vi "Discrete Integrator (DBL Array).vi"(2 "initialize":bool, 3 "initial conditions":dbl[](array[numeric]) format="%.2f", 5 "input points":dbl[](array[numeric]) format="%.2f") -> (1 "output points":dbl[](array[numeric]) format="%.2f")   [LabVIEW 2017, in "NI_AdvCtrl_discrete linear.lvlib"]
doc: "LabVIEW no longer supports this VI. You can obtain similar functionality by installing the LabVIEW Simulation Module.\n\nIntegrates a discrete input signal. The integration process is based on Euler method."
uses:
  <vilib>/addons/control/advanced/NI_AdvCtrl_discrete linear.lvlib
  <vilib>/addons/control/advanced/NI_AdvCtrl_continuous linear.lvlib
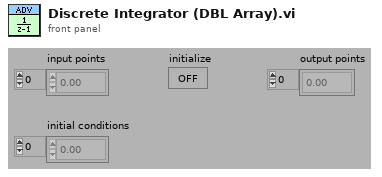
[diagram p1: front panel]
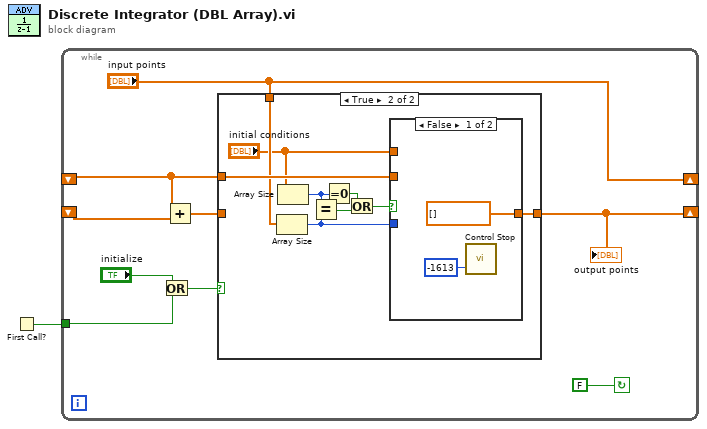
[diagram p0: block diagram]
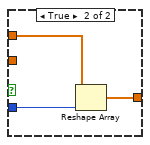
[diagram p3: hidden frame]
diagram:
  n1 = First Call?() -> (First Call?: T/F=w1:bool)
  n2 = while {
    shift-left: _ -> [w3]
    shift-right: ["input points"] -> _
    tunnel: w1 -> [w8]
    shift-left: _ -> [w6]
    shift-right: [w4] -> _
    stop <- FALSE continue-if-true
    n3 = Or(x="initialize", y=w8) -> (x .or. y?=w7:bool)
    n4 = Add(x=w3, y=w6) -> (x+y=w5:dbl[])
    n5 = case shown="True" w7 {
      tunnel: w3 -> [_ w20]
      tunnel: [w11 w19] -> w4
      tunnel: w5 -> [w11 _]
      tunnel: "input points" -> [_ w18]
      frame False {
      }
      frame True {
        n6 = Array Size(array=w18) -> (size(s)=w15:i32)
        n7 = Array Size(array="initial conditions") -> (size(s)=w13:i32)
        n8 = Equal?(x=w13, y=w15) -> (x = y?=w16:bool)
        n9 = Equal To 0?(x=w13) -> (x = 0?=w12:bool)
        n10 = Or(x=w12, y=w16) -> (x .or. y?=w14:bool)
        n11 = case shown="False" w14 {
          tunnel: w20 -> [_ _]
          tunnel: [dbl[] [] ("Initial Values") w24] -> w19
          tunnel: "initial conditions" -> [_ w25]
          tunnel: w15 -> [_ w23]
          frame False {
            n12 = call <vilib>:"Control Stop.vi"("error"=-1613) -> ()  [unwired: 2 out]
          }
          frame True {
            n13 = Reshape Array(w25, w23) -> (w24:dbl[])
          }
        }
      }
    }
    "output points" <- w4
  }
